vi "Platform 수신.vi"() -> (0 "Platform error out":errorcluster caption="error out")   [LabVIEW 2016]
panel:
  in  "stop?":bool
  in  "Platform error in":errorcluster
  in  "Platform Baud rate":u32(ring)=115200 items=["Auto Connect"=0, "300"=300, "600"=600, "1200"=1200, "2400"=2400, "4800"=4800, "9600"=9600, "19200"=19200, "38400"=38400, "57600"=57600, "115200"=115200]
  out "Encoder_distance":dbl
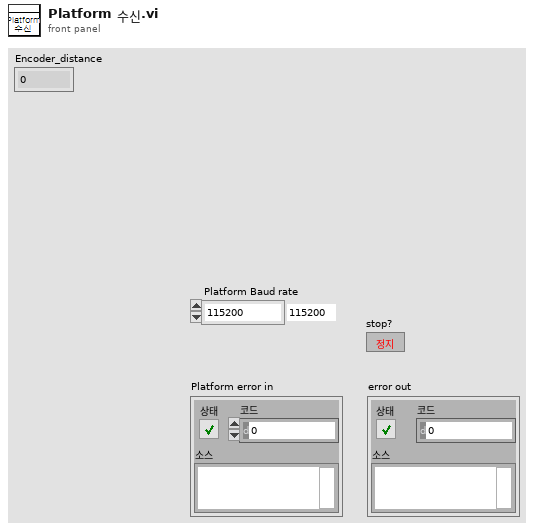
[diagram p1: front panel]
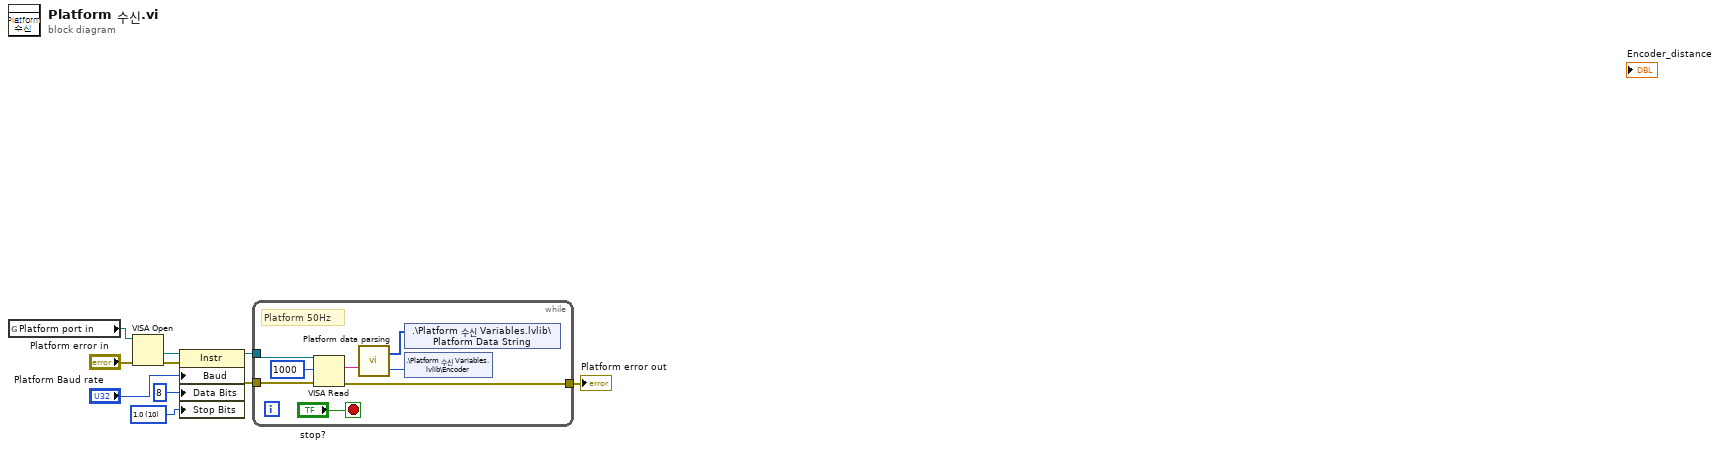
[diagram p0: block diagram]
diagram:
  w9 = u16 10 items=["1.0"=10, "1.5"=15, "2.0"=20] ("Serial Settings:Stop Bits")
  n1 = global read "[GV]_PLATFORM Port NUM.vi" "Platform port in"() -> (w1:refnum<visa-resource-name>)
  n2 = VISA Open(error in (no error)="Platform error in", VISA resource name=w1) -> (VISA resource name=w8:refnum<visa-resource-name>, error out=w6:errorcluster)  [unwired: 3 in]
  n3 = property class="Instr"(reference=w8, error in=w6, "Baud"="Platform Baud rate", "Data Bits"=u16 8 ("Serial Settings:Data Bits"), "Stop Bits"=w9) -> (reference out=w4:refnum<visa-resource-name>, error out=w3:errorcluster)
  n4 = while {
    tunnel: w4 -> [w16]
    tunnel: w3 -> [w18]
    tunnel: [w15] -> w2
    stop <- "stop?" stop-if-true
    # "Platform 50Hz"
    n5 = VISA Read(VISA resource name=w16, byte count=u32 1000 ("바이트 카운트"), error in (no error)=w18) -> (read buffer=w13:string, error out=w15:errorcluster)  [unwired: 2 out]
    n6 = call "Platform data parsing.vi"("Platform Data"=w13) -> ("Encoder"=w12:i64, "Platform Data Array"=w11:i64[])  [unwired: 2 in]
    n7 = shared-variable ".\\Platform 수신 Variables.lvlib\\Platform Data String"(w11) -> ()  [unwired: 1 in, 1 out]
    n8 = shared-variable ".\\Platform 수신 Variables.lvlib\\Encoder"(w12) -> ()  [unwired: 1 in, 1 out]
  }
  "Platform error out" <- w2
